vi "总磷总氮启动参数对话框.vi"() -> (2 "确认":bool, 3 "元素":cluster{"命令":string, "data":variant})   [LabVIEW 2016, in "斯坦道总磷总氮V2.lvlib"]
panel:
  out "标液值":dbl caption="标液值："
  in  "取消":bool
  in  "确定":bool
  in  "量程切换":u16(ring)=2 items=["高量程", "低量程", "自动"]
  in  "站号":u16(ring)=1 items=["氨氮"=3]
  in  "控制命令":T1(ring)
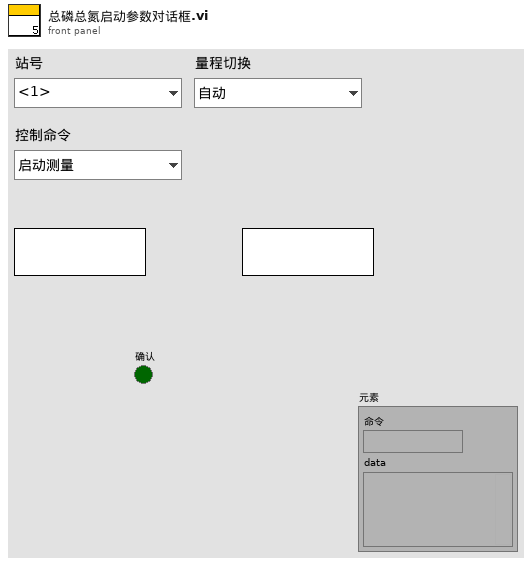
[diagram p1: front panel]
types:
  T1 = enum16{"启动测量", "标样核查", "零点核查", "跨度核查", "空白测试", "平行样测试", "加标回收", "空白校准", "标样校准", "初始化（清洗）", "停止测试", "仪器重启", "校时", "模式设置", "测量间隔设置"}
  T2 = typedef "LVStringsAndValuesArrayTypeDef_U16.ctl" = cluster{"String":string, "Value":u16}[]
  T3 = cluster{"站号":u16, "量程切换":enum32{"H", "L", "AUTO"}, "控制命令":enum16{"启动测量", "标样核查", "零点核查", "跨度核查", "空白测试", "平行样测试", "加标回收", "空白校准", "标样校准", "初始化（清洗）", "停止测试", "仪器重启", "校时", "模式设置", "测量间隔设置", "盲样测试"}, "模式设置":enum16{"待机", "连续模式", "周期模式", "定点模式", "受控模式", "手动模式"}, "测量间隔":u16}
  T4 = cluster{"总磷跨度值":dbl, "总磷零点标准液浓度":dbl, "总磷跨度标准液浓度":dbl, "总磷标准液标准浓度":dbl, "总氮跨度值":dbl, "总氮零点标准液浓度":dbl, "总氮跨度标准液浓度":dbl, "总氮标准液标准浓度":dbl, "COD跨度值":dbl, "COD零点标准液浓度":dbl, "COD跨度标准液浓度":dbl, "COD标准液标准浓度":dbl, "氨氮跨度值":dbl, "氨氮零点标准液浓度":dbl, "氨氮跨度标准液浓度":dbl, "氨氮标准液标准浓度":dbl, "磷酸盐跨度值":dbl, "磷酸盐零点标准液浓度":dbl, "磷酸盐跨度标准液浓度":dbl, "磷酸盐标准液标准浓度":dbl, "硝氮跨度值":dbl, "硝氮零点标准液浓度":dbl, "硝氮跨度标准液浓度":dbl, "硝氮标准液标准浓度":dbl, "亚硝氮跨度值":dbl, "亚硝氮零点标准液浓度":dbl, "亚硝氮跨度标准液浓度":dbl, "亚硝氮标准液标准浓度":dbl, "硫化物跨度值":dbl, "硫化物零点标准液浓度":dbl, "硫化物跨度标准液浓度":dbl, "硫化物标准液标准浓度":dbl, "硅酸盐跨度值":dbl, "硅酸盐零点标准液浓度":dbl, "硅酸盐跨度标准液浓度":dbl, "硅酸盐标准液标准浓度":dbl}
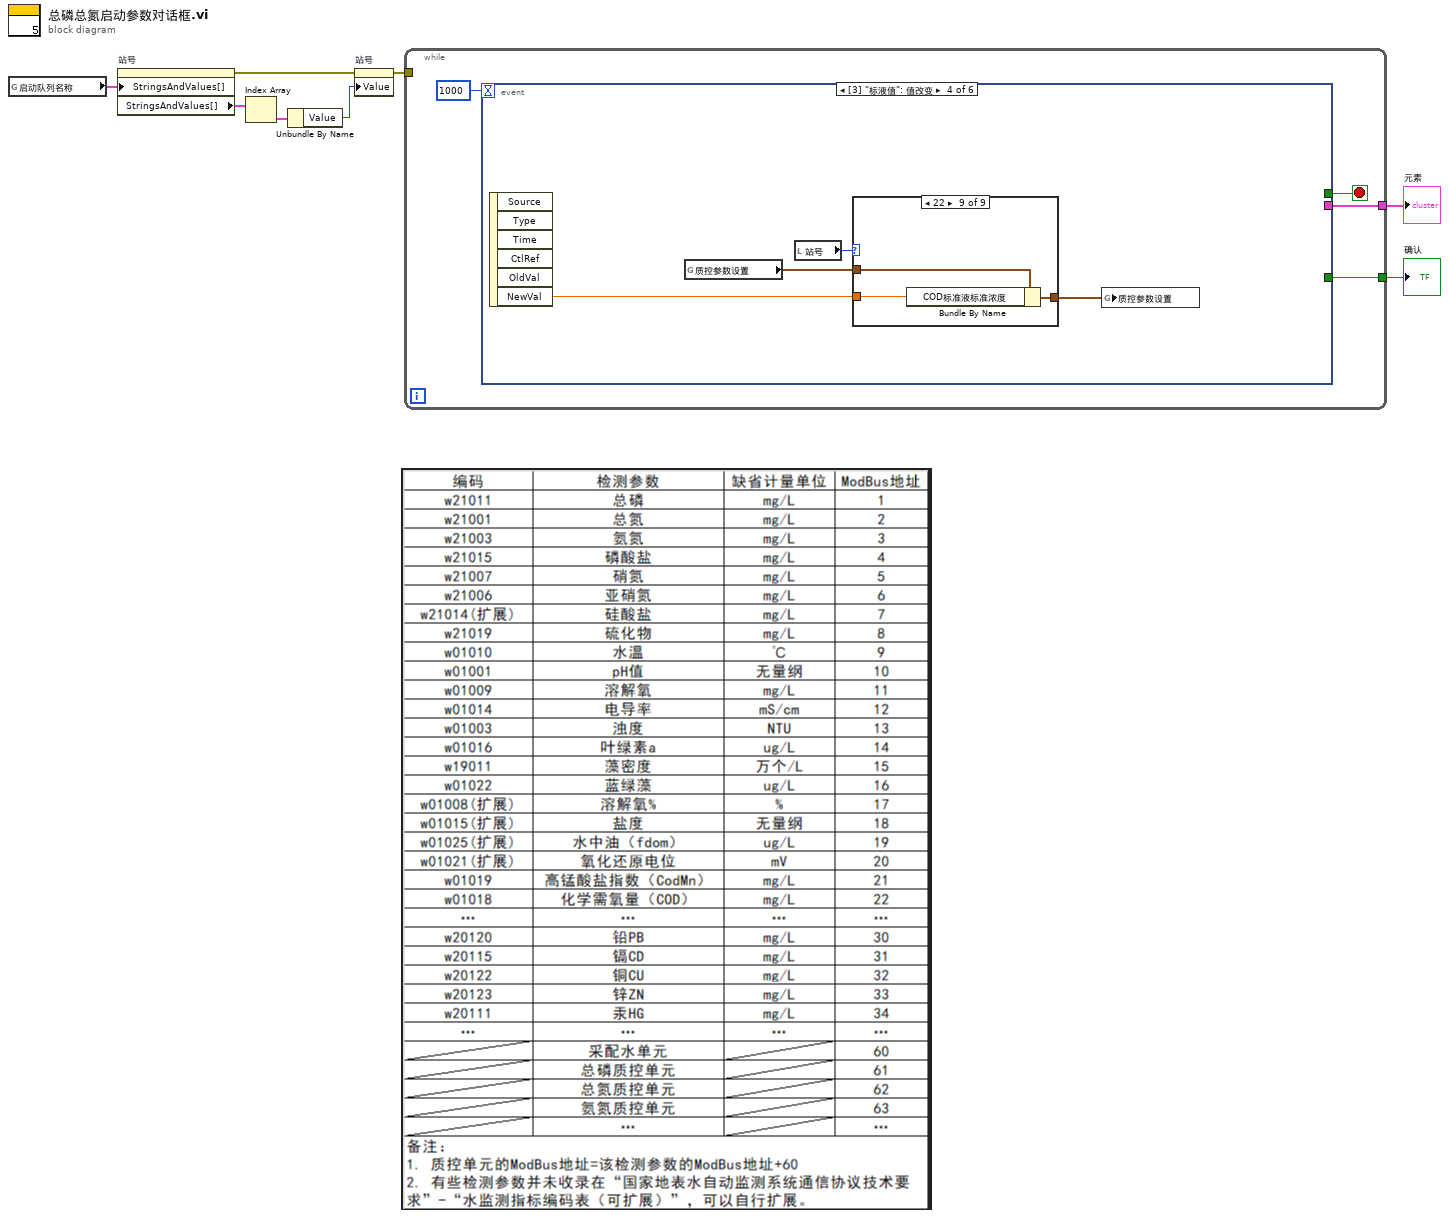
[diagram p0: block diagram]
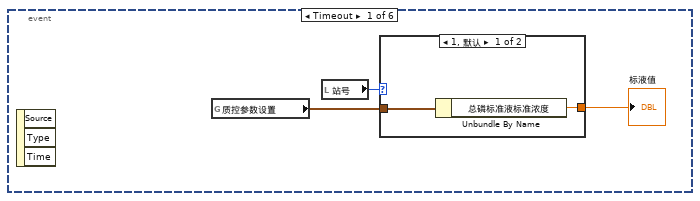
[diagram p2: hidden frame]
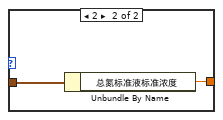
[diagram p3: hidden frame]
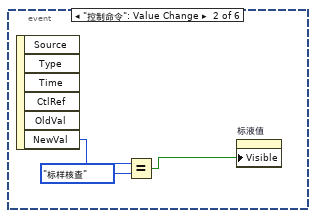
[diagram p4: hidden frame]
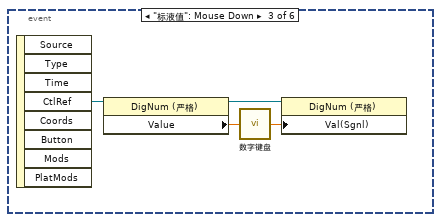
[diagram p5: hidden frame]
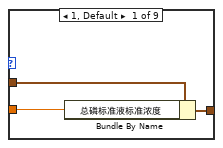
[diagram p6: hidden frame]
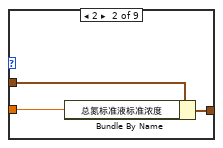
[diagram p7: hidden frame]
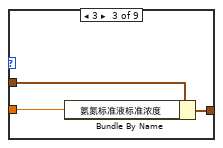
[diagram p8: hidden frame]
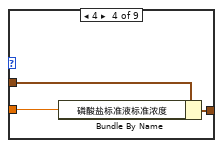
[diagram p9: hidden frame]
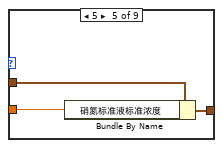
[diagram p10: hidden frame]
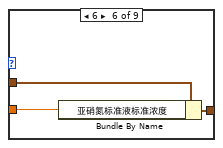
[diagram p11: hidden frame]
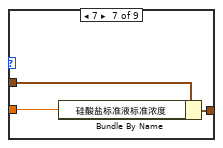
[diagram p12: hidden frame]
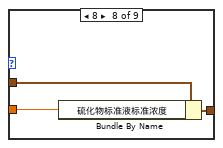
[diagram p13: hidden frame]
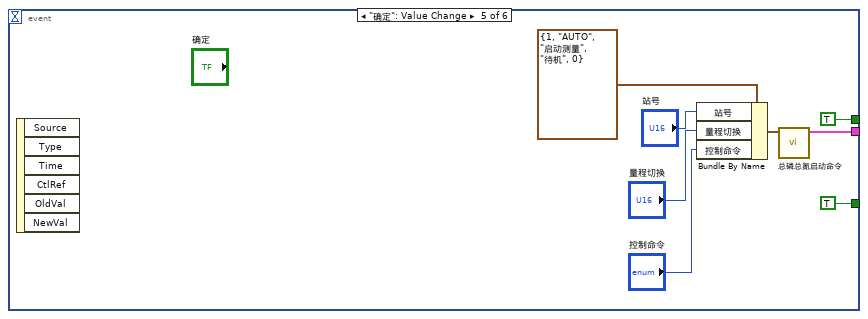
[diagram p14: hidden frame]
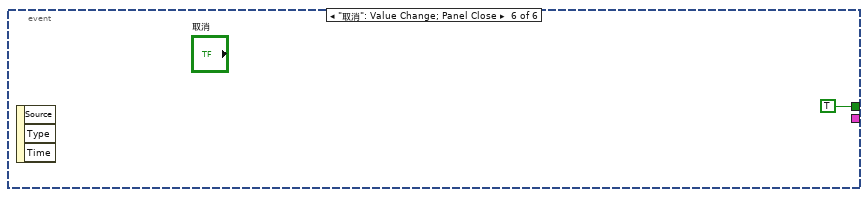
[diagram p15: hidden frame]
diagram:
  n1 = global read "总磷总氮断电保存全局变量.vi" "启动队列名称"() -> (w6:cluster{"String":string, "Value":u16}[])
  n2 = property on="站号" class="Ring (严格)"("StringsAndValues[]"=w6) -> (error out=w5:errorcluster, "StringsAndValues[]"=w4:T2)  [unwired: 2 in, 1 out]
  n3 = Index Array(array=w4) -> (element=w3:cluster{"String":string, "Value":u16})  [unwired: 1 in]
  n4 = Unbundle By Name(w3) -> ("Value"=w2:u16)
  n5 = property on="站号" class="Ring (严格)"(error in=w5, "Value"=w2) -> (error out=w1:errorcluster)  [unwired: 1 in, 1 out]
  n6 = while {
    tunnel: [w10] -> w8
    tunnel: [w9] -> w7
    tunnel: w1 -> [_]
    stop <- w12 stop-if-true
    n7 = event shown="[3] \"标液值\": 值改变" {
      selector: _ -> [_ _ _ _ _ _]
      dyn-events: _ -> [_ _ _ _ _ _]
      timeout: 1000 -> [_ _ _ _ _ _]
      tunnel: [_ _ _ _ TRUE TRUE] -> w12
      tunnel: [_ _ _ _ TRUE _] -> w10
      tunnel: [_ _ _ _ w63 _] -> w9
      event Timeout {
        n8 = event-data() -> ()  [unwired: 1 in, 3 out]
        n9 = global read "总磷总氮断电保存全局变量.vi" "质控参数设置"() -> (w15:T4)
        n10 = local read "站号"() -> (w14:u16)
        n11 = case shown="1, 默认" w14 {
          tunnel: w15 -> [w17 w19]
          tunnel: [w16 w18] -> w13
          frame 1, Default {
            n12 = Unbundle By Name(w17) -> ("总磷标准液标准浓度"=w16:dbl)
          }
          frame 2 {
            n13 = Unbundle By Name(w19) -> ("总氮标准液标准浓度"=w18:dbl)
          }
        }
        "标液值" <- w13
      }
      event "控制命令": Value Change {
        n14 = event-data() -> ("NewVal"=w22:T1)  [unwired: 1 in, 5 out]
        n15 = Equal?(x=w22, y=T1."标样核查") -> (x = y?=w20:bool)
        n16 = property on="标液值" class="DigNum (严格)"("Visible"=w20) -> ()  [unwired: 2 in, 2 out]
      }
      event "标液值": Mouse Down {
        n17 = event-data() -> ("CtlRef"=w26:refnum<vi>)  [unwired: 1 in, 7 out]
        n18 = property class="DigNum (严格)"(reference=w26) -> (reference out=w23:refnum<vi>, "Value"=w25:dbl)  [unwired: 1 in, 1 out]
        n19 = call "数字键盘.vi"("OldNumber"=w25) -> ("NewNumber"=w24:dbl)
        n20 = property class="DigNum (严格)"(reference=w23, "Val(Sgnl)"=w24) -> ()  [unwired: 1 in, 2 out]
      }
      event "标液值": Value Change {
        n21 = event-data() -> ("NewVal"=w28:dbl)  [unwired: 1 in, 5 out]
        n22 = global read "总磷总氮断电保存全局变量.vi" "质控参数设置"() -> (w29:T4)
        n23 = local read "站号"() -> (w30:u16)
        n24 = case shown="22" w30 {
          tunnel: w29 -> [w33 w36 w39 w42 w45 w48 w51 w54 w57]
          tunnel: [w31 w34 w37 w40 w43 w46 w49 w52 w55] -> w27
          tunnel: w28 -> [w32 w35 w38 w41 w44 w47 w50 w53 w56]
          frame 1, Default {
            n25 = Bundle By Name(cluster=w33, "总磷标准液标准浓度"=w32) -> (w31:T4)
          }
          frame 2 {
            n26 = Bundle By Name(cluster=w36, "总氮标准液标准浓度"=w35) -> (w34:T4)
          }
          frame 3 {
            n27 = Bundle By Name(cluster=w39, "氨氮标准液标准浓度"=w38) -> (w37:T4)
          }
          frame 4 {
            n28 = Bundle By Name(cluster=w42, "磷酸盐标准液标准浓度"=w41) -> (w40:T4)
          }
          frame 5 {
            n29 = Bundle By Name(cluster=w45, "硝氮标准液标准浓度"=w44) -> (w43:T4)
          }
          frame 6 {
            n30 = Bundle By Name(cluster=w48, "亚硝氮标准液标准浓度"=w47) -> (w46:T4)
          }
          frame 7 {
            n31 = Bundle By Name(cluster=w51, "硅酸盐标准液标准浓度"=w50) -> (w49:T4)
          }
          frame 8 {
            n32 = Bundle By Name(cluster=w54, "硫化物标准液标准浓度"=w53) -> (w52:T4)
          }
          frame 22 {
            n33 = Bundle By Name(cluster=w57, "COD标准液标准浓度"=w56) -> (w55:T4)
          }
        }
        n34 = global write "总磷总氮断电保存全局变量.vi" "质控参数设置"(w27) -> ()
      }
      event "确定": Value Change {
        n35 = event-data() -> ()  [unwired: 1 in, 6 out]
        n36 = Bundle By Name(cluster=T3 {"站号"=1, "量程切换"=enum."AUTO", "控制命令"=enum."启动测量", "模式设置"=enum."待机", "测量间隔"=0} ("参数"), "站号"="站号", "量程切换"="量程切换", "控制命令"="控制命令") -> (w61:T3)
        n37 = call "总磷总氮启动命令.vi"("参数"=w61) -> ("启动命令"=w63:cluster{"命令":string, "data":variant})  [unwired: 10 in]
      }
      event "取消": Value Change; Panel Close {
        n38 = event-data() -> ()  [unwired: 1 in, 3 out]
      }
    }
  }
  "元素" <- w7
  "确认" <- w8
